vi "FL_Make_data_frame_and_put_to_queue.vi"(8 "error in":errorcluster, 10 "Queue in":refnum<queue>, 11 "VISA resource name in":refnum<visa-resource-name>) -> (0 "error out":errorcluster, 1 "Timestamp":timestamp, 2 "Queue out":refnum<queue>, 3 "VISA resource name out":refnum<visa-resource-name>, 5 "Read buffer (for reference only, data is queued)":string)   [LabVIEW 2018, in "Tracker.lvlib"]
uses:
  Tracker.lvlib
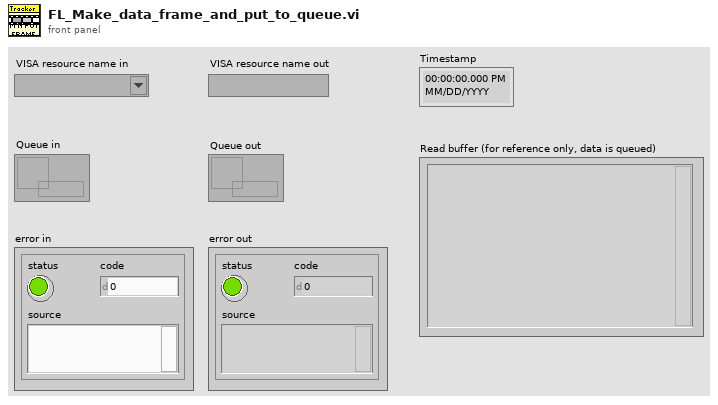
[diagram p1: front panel]
types:
  T1 = cluster{string, "seconds since 1Jan1904":timestamp}
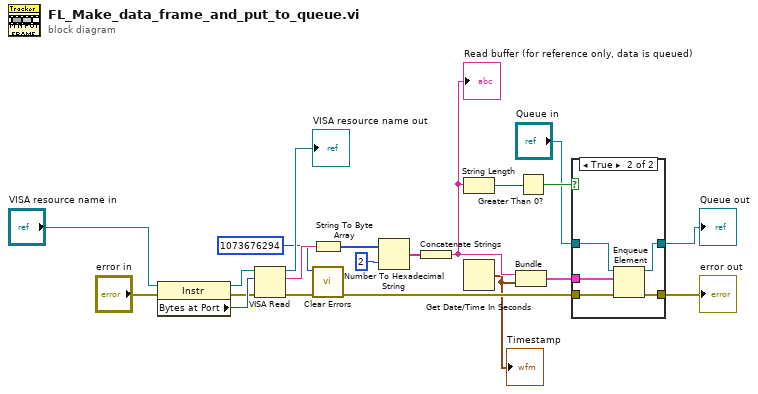
[diagram p0: block diagram]
diagram:
  n1 = property class="Instr"(reference="VISA resource name in", error in="error in") -> (reference out=w5:refnum<visa-resource-name>, error out=w6:errorcluster, "Bytes at Port"=w7:u32)
  n2 = VISA Read(VISA resource name=w5, byte count=w7, error in (no error)=w6) -> (VISA resource name out=→"VISA resource name out":refnum<visa-resource-name>, read buffer=w9:string, error out=w10:errorcluster)  [unwired: 1 out]
  n3 = String To Byte Array(string=w9) -> (unsigned byte array=w1:u8[])
  n4 = call <vilib>:"Clear Errors.vi"("error in (no error)"=w10, "specific error code to clear (0: all)"=1073676294) -> ("error out"=w19:errorcluster)  [unwired: 4 in, 1 out]
  n5 = Number To Hexadecimal String(1:i16 2 ("width (-)"), 2:w1) -> (0:w3:string[])
  n6 = Concatenate Strings(w3) -> (w21:string)
  "Read buffer (for reference only, data is queued)" <- w21
  n7 = String Length(string=w21) -> (length=w15:i32)
  n8 = Get Date/Time In Seconds ("Current time")() -> (seconds since 1Jan1904=w14:timestamp)
  "Timestamp" <- w14
  n9 = Bundle(w21, "seconds since 1Jan1904"=w14) -> (w18:T1)  [unwired: 1 in]
  n10 = Greater Than 0?(x=w15) -> (x > 0?=w20:bool)
  n11 = case shown="True" w20 {
    tunnel: w18 -> [_ w24]
    tunnel: w19 -> [w23 w26]
    tunnel: [w23 w25] -> w11
    tunnel: "Queue in" -> [w22 w28]
    tunnel: [w22 w27] -> w13
    frame False {
    }
    frame True {
      n12 = Enqueue Element(queue=w28, element=w24, error in (no error)=w26) -> (queue out=w27:refnum<queue>, error out=w25:errorcluster)  [unwired: 1 in, 1 out]
    }
  }
  "Queue out" <- w13
  "error out" <- w11
